vi "TouchMux.vi"(2 "NXT":T2={"Hardware"="NXT", "Flattened String"=""}, 3 "Input Port":T1 items=["Port 1", "Port 2", "Port 3", "Port 4"]) -> (1 "Touch Mux Output":i16 caption="Scaled Value", 4 "NXT dup":T2={"Hardware"="NXT", "Flattened String"=""} caption="NXT")   [LabVIEW 2010]
uses:
  <vilib>/NXT/Subs/LVHSConnector.ctl
  <vilib>/NXT/Block Support/NXT_InputPort.ctl
  <vilib>/NXT/Block Support/HWPage.SensorType.ctl
  <vilib>/NXT/Block Support/HWPage.SensorMode.ctl
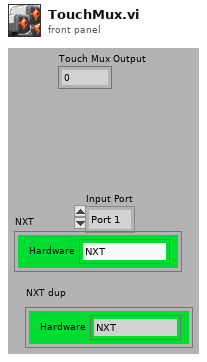
[diagram p1: front panel]
types:
  T1 = typedef "NXT_InputPort.ctl" = u8
  T2 = typedef "LVHSConnector.ctl" = cluster{"Hardware":string, "Flattened String":string}
  T3 = typedef "HWPage.SensorType.ctl" = u8
  T4 = typedef "HWPage.SensorMode.ctl" = u8
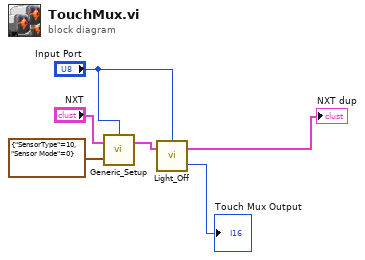
[diagram p0: block diagram]
diagram:
  n1 = call <vilib>:"Generic_Setup.vi"("Sensor Setup"=cluster{"SensorType":T3, "Sensor Mode":T4} {"SensorType"=10, "Sensor Mode"=0}, "NXT"="NXT", "Port"="Input Port") -> ("NXT"=w2:T2)  [unwired: 1 out]
  n2 = call <vilib>:"Light_Off.vi"("NXT"=w2, "Port (Port 3)"="Input Port") -> ("Scaled Value"=→"Touch Mux Output":i16, "NXT"=→"NXT dup":T2)  [unwired: 1 in]
